vi "Execute.vi"(8 "error in":errorcluster, 11 "Wait in":refnum<class "Wait.lvclass">) -> (0 "error out":errorcluster, 1 "Next Step?":bool, 2 "MSG":string, 3 "Wait out":refnum<class "Wait.lvclass">)   [LabVIEW 2015, in "Wait.lvclass"]
uses:
  Wait.lvclass
  Wait.lvclass/Wait.ctl
  Reusable/Sequence/STEPS/STEP.lvclass/STEP.ctl
  Read Wait Time.vi
  Reusable/Sequence/STEPS/Read First Call.vi
  Reusable/Sequence/STEPS/Write First Call.vi
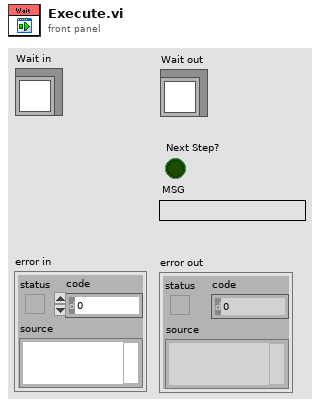
[diagram p1: front panel]
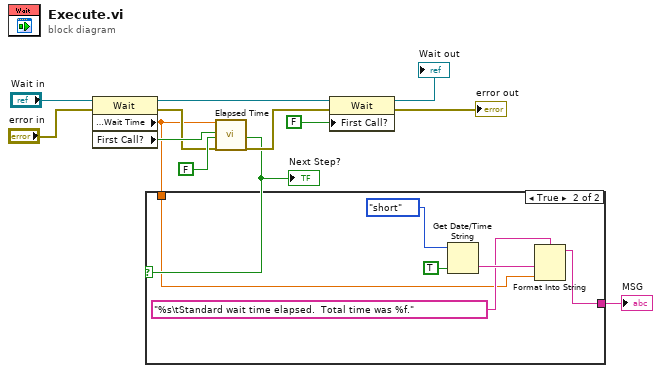
[diagram p0: block diagram]
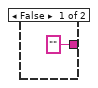
[diagram p2: hidden frame]
diagram:
  n1 = property class="Wait"(reference="Wait in", error in="error in") -> (reference out=w12:refnum<class "Wait.lvclass">, error out=w6:errorcluster, "Data Access:Wait Time"=w1:dbl, "First Call?"=w9:bool)
  n2 = call "Elapsed Time"("Time Target (s)"=w1, "Reset"=w9, "Auto Reset"=FALSE, "error in (no error)"=w6) -> ("Time has Elapsed"=w3:bool, "error out"=w5:errorcluster)  [unwired: 8 in, 6 out]
  "Next Step?" <- w3
  n3 = case shown="True" w3 {
    tunnel: ["" w15] -> w2
    tunnel: w1 -> [_ w16]
    frame False {
    }
    frame True {
      n4 = Get Date/Time String(date format (0)=enum16{"short", "long", "abbreviated"}."short", want seconds? (F)=TRUE) -> (time string=w18:string)  [unwired: 1 in, 1 out]
      n5 = Format Into String(format string="%s\tStandard wait time elapsed.  Total time was %f.", w18, w16) -> (resulting string=w15:string)  [unwired: 2 in, 1 out]
    }
  }
  "MSG" <- w2
  n6 = property class="Wait"(reference=w12, error in=w5, "First Call?"=FALSE) -> (reference out=→"Wait out":refnum<class "Wait.lvclass">, error out=→"error out":errorcluster)
